vi "RT Main.vi"() -> ()   [LabVIEW 2015]
doc: "The top-level VI for the RIO Eval Kit.\n\nThis VI runs through multiple stages. Each stage demonstrates different features of the RIO Eval Kit. The program uses a \"Queued Message Handler\" architecture. The top loop reads and writes information to and from the FPGA. That information is sent to the bottom through a queue. The information being transfered includes both the data and the type of message being sent. The bottom loop then handles displaying the appropriate information on the LCD."
uses:
  controls/SystemStates.ctl
  <vilib>/EmbeddedDisplay/Hitachi HD44780/Common/Control/screen size.ctl
  <vilib>/EmbeddedDisplay/Hitachi HD44780/Common/Control/font configuration.ctl
  controls/Queue Data.ctl
  controls/SoundOptions.ctl
  <vilib>/FPGAPlugInAG/sbRIO-9637/niLvFpga_Open_sbRIO-9637.vi
  <vilib>/rvi/interface/common/dynamic/niFpgaDynamicAddResources.vi
  <vilib>/Utility/error.llb/Error Cluster From Error Code.vi
  <vilib>/rvi/errors/niLvFpgaAdjustHostInterfaceError.vi
  <vilib>/FPGAPlugInAG/Dynamic/niLvFpga_Close_Dynamic.vi
  <vilib>/rvi/interface/nirviOpenFPGA/nirviOpenFPGA.xnode
  FPGA Bitfiles/LabVIEWRIOEvalua_FPGATarget_FPGA_fRdPegB0rcM.lvbitx
  <vilib>/rvi/interface/nirviMethod/nirviMethod.xnode
  <vilib>/rvi/interface/nirviReadWriteControl/nirviReadWriteControl.xnode
  <vilib>/rvi/interface/nirviCloseFPGA/nirviCloseFPGA.xnode
  <vilib>/EmbeddedDisplay/Hitachi HD44780/Host/HD44780 Host.lvlib
  <vilib>/EmbeddedDisplay/Hitachi HD44780/Common/HD44780 Common.lvlib
  NiFpgaLv.dll
  <vilib>/rvi/interface/Simulation/niFpgaSimulationCallBeginRW.vi
  <vilib>/FPGAPlugInAG/Dynamic/niLvFpga_ReadFifo_Dynamic.vi
  <vilib>/rvi/errors/niLvFpgaMergeErrorWithErrorCode.vi
  usr/local/lib/libamplitude.dll
panel:
  out "Signal":dbl[](graph)
  out "Alarm":bool
  in  "Alarm Threshold":dbl=4.0
  out "Amplitude":dbl format="%#_3g"
  # "Start by turning encoder right to kickoff first stage, and \ncontinue turning right to complete all three stages. Stop \nthe program at any time by pressing the right button (PB2)."
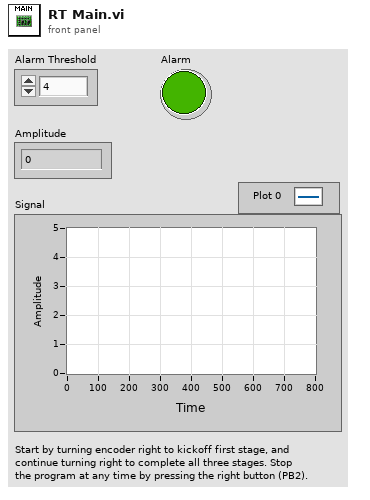
[diagram p1: front panel]
types:
  T1 = typedef "Queue Data.ctl" = cluster{"Current Pos > Threshold?":bool, "Current Pos > Previous?":bool, "Amplitude":dbl, "Stage Number":string}
  T2 = typedef "HD44780 Common.lvlib/font configuration.ctl" = enum8{"5x8 & 2 lines", "5x10 & 1 line", "5x8 & 1 line"}
  T3 = typedef "HD44780 Common.lvlib/screen size.ctl" = enum8{"8x1", "8x2", "12x4", "16x1", "16x2", "16x4", "20x1", "20x2", "20x4", "24x1", "24x2", "40x2", "40x4"}
  T4 = typedef "SystemStates.ctl" = enum16{"Shutdown", "Stage 1", "Stage 2", "Stage 3", "Alarm State"}
  T5 = typedef "SoundOptions.ctl" = enum16{"Ding", "Boing", "Buzzer", "Horn"}
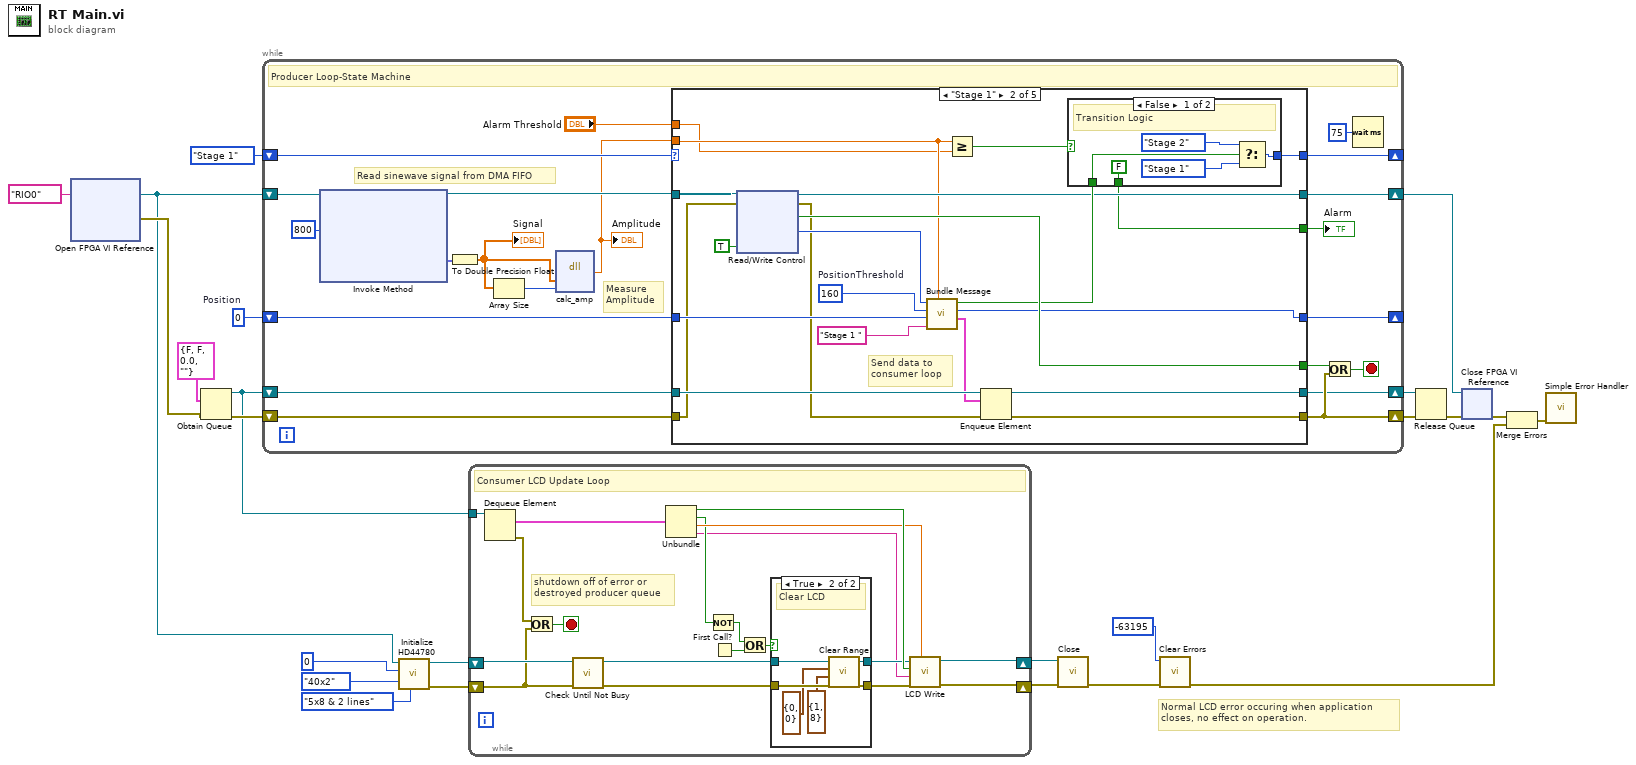
[diagram p0: block diagram]
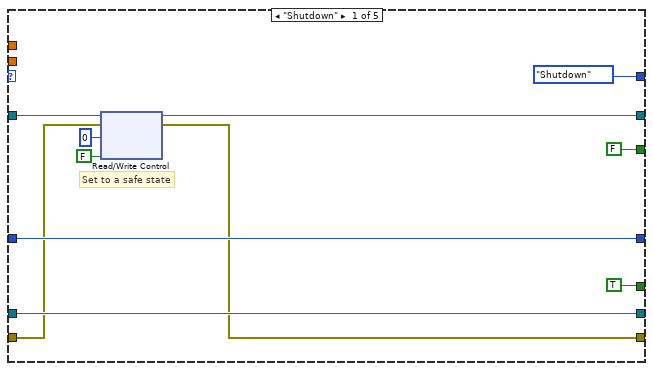
[diagram p3: hidden frame]
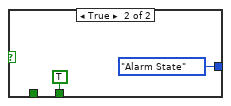
[diagram p4: hidden frame]
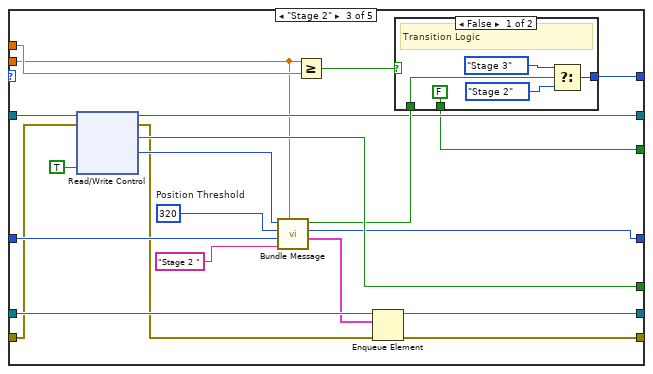
[diagram p5: hidden frame]
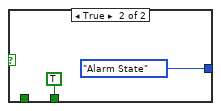
[diagram p6: hidden frame]
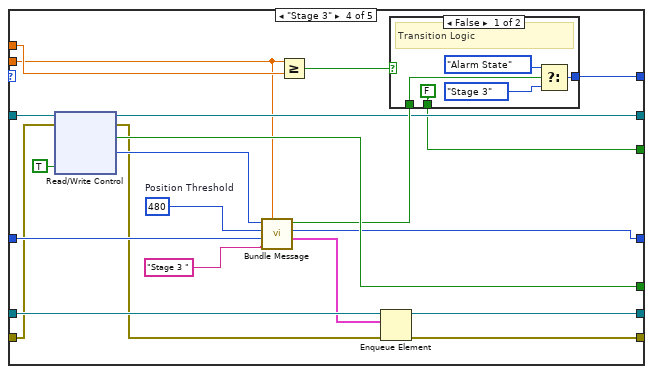
[diagram p7: hidden frame]
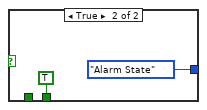
[diagram p8: hidden frame]
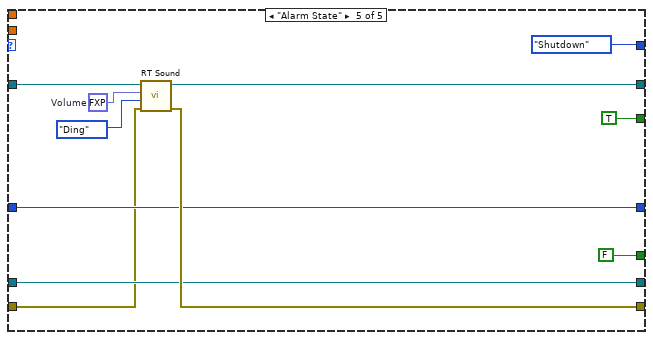
[diagram p9: hidden frame]
diagram:
  w4 = i16 0  # Position
  # "Normal LCD error occuring when application\ncloses, no effect on operation."
  n1 = xnode "Open FPGA VI Reference"("resource name"=tag "RIO0") -> ("FPGA VI Reference Out"=w6:refnum<k20>, "error out"=w10:errorcluster)  [unwired: 1 in]
  n2 = Obtain Queue(element data type=T1 {"Current Pos > Threshold?"=FALSE, "Current Pos > Previous?"=FALSE, "Amplitude"=0.0, "Stage Number"=""} ("output to queue"), error in (no error)=w10) -> (queue out=w7:refnum<queue>, error out=w9:errorcluster)  [unwired: 3 in, 1 out]
  n3 = while {
    shift-right: [w39] -> w23
    shift-left: w9 -> [w28]
    shift-right: [w37] -> w24
    shift-left: w7 -> [w45]
    shift-right: [w41] -> _
    shift-left: SystemStates."Stage 1" ("Enum") -> [w42]
    shift-right: [w29] -> _
    shift-left: w4 -> [w40]
    shift-right: [w36] -> w5
    shift-left: w6 -> [w34]
    stop <- w43 stop-if-true
    # "Measure\nAmplitude"
    # "Read sinewave signal from DMA FIFO"
    # "Producer Loop-State Machine"
    n4 = xnode "Invoke Method"("FPGA VI Reference In"=w34, "Number of Elements"=u32 800) -> ("FPGA VI Reference Out"=w32:refnum<k20>, "Data"=w35:fxp<+/-,24,5>[])  [unwired: 2 in, 2 out]
    n5 = To Double Precision Float(number=w35) -> (double precision float=w26:dbl[])
    "Signal" <- w26
    n6 = Array Size(array=w26) -> (size(s)=w27:i32)
    n7 = dll-call lib="usr/local/lib/libamplitude.*" fn="calc_amp"("waveform"=w26, "length"=w27) -> ("return type"=w25:dbl)  [unwired: 5 in, 2 out]
    "Amplitude" <- w25
    n8 = case shown="\"Stage 1\"" w42 {
      tunnel: w45 -> [w49 w77 w105 w133 w147]
      tunnel: [w48 w76 w104 w132 w151] -> w39
      tunnel: [TRUE w75 w103 w131 FALSE ("E-Stop")] -> w38
      tunnel: [SystemStates."Shutdown" ("Enum") w74 w102 w130 SystemStates."Shutdown" ("Enum")] -> w41
      tunnel: w40 -> [w50 w61 w89 w117 w143]
      tunnel: [w49 w68 w96 w124 w147] -> w37
      tunnel: w32 -> [w53 w67 w95 w123 w142]
      tunnel: [w52 w66 w94 w122 w146] -> w36
      tunnel: w25 -> [_ w63 w92 w120 _]
      tunnel: [FALSE w64 w90 w118 TRUE] -> w31
      tunnel: "Alarm Threshold" -> [_ w62 w93 w121 _]
      tunnel: [w50 w60 w88 w116 w143] -> w29
      tunnel: w28 -> [w47 w57 w85 w113 w141]
      frame "Shutdown" {
        # "Set to a safe state"
        n9 = xnode "Read/Write Control"("FPGA VI Reference In"=w53, "error in"=w47, "Position"=i16 0, "PWM"=FALSE) -> ("FPGA VI Reference Out"=w52:refnum<k20>, "error out"=w48:errorcluster)
      }
      frame "Stage 1" {
        w70 = i16 160  # PositionThreshold
        # "Send data to\nconsumer loop"
        n10 = xnode "Read/Write Control"("FPGA VI Reference In"=w67, "error in"=w57, "PWM"=TRUE) -> ("FPGA VI Reference Out"=w66:refnum<k20>, "error out"=w58:errorcluster, "E-Stop"=w75:bool, "Position"=w69:i16)
        n11 = call "Bundle Message.vi"("Amplitude"=w63, "Stage Number"="Stage 1 " ("text"), "Previous Position"=w61, "Position Threshold"=w70, "Current Position"=w69) -> ("Output to queue"=w59:T1, "Output Position"=w60:i16, "Transition?"=w72:bool)  [unwired: 4 in]
        n12 = Greater Or Equal?(x=w63, y=w62) -> (x >= y?=w65:bool)
        n13 = Enqueue Element(queue=w77, element=w59, error in (no error)=w58) -> (queue out=w68:refnum<queue>, error out=w76:errorcluster)  [unwired: 1 in, 1 out]
        n14 = case shown="False" w65 {
          tunnel: [w80 SystemStates."Alarm State" ("Enum")] -> w74
          tunnel: w72 -> [w79 _]
          tunnel: [FALSE TRUE] -> w64
          frame False {
            # "Transition Logic"
            n15 = Select(t=SystemStates."Stage 2" ("Enum"), s=w79, f=SystemStates."Stage 1" ("Enum")) -> (s? t:f=w80:T4)
          }
          frame True {
          }
        }
      }
      frame "Stage 2" {
        w98 = i16 320  # Position Threshold
        n16 = xnode "Read/Write Control"("FPGA VI Reference In"=w95, "error in"=w85, "PWM"=TRUE) -> ("FPGA VI Reference Out"=w94:refnum<k20>, "error out"=w86:errorcluster, "E-Stop"=w103:bool, "Position"=w97:i16)
        n17 = call "Bundle Message.vi"("Amplitude"=w92, "Stage Number"="Stage 2 " ("text"), "Previous Position"=w89, "Position Threshold"=w98, "Current Position"=w97) -> ("Output to queue"=w87:T1, "Output Position"=w88:i16, "Transition?"=w99:bool)  [unwired: 4 in]
        n18 = Greater Or Equal?(x=w92, y=w93) -> (x >= y?=w91:bool)
        n19 = Enqueue Element(queue=w105, element=w87, error in (no error)=w86) -> (queue out=w96:refnum<queue>, error out=w104:errorcluster)  [unwired: 1 in, 1 out]
        n20 = case shown="False" w91 {
          tunnel: [w108 SystemStates."Alarm State" ("Enum")] -> w102
          tunnel: w99 -> [w107 _]
          tunnel: [FALSE TRUE] -> w90
          frame False {
            # "Transition Logic"
            n21 = Select(t=SystemStates."Stage 3" ("Enum"), s=w107, f=SystemStates."Stage 2" ("Enum")) -> (s? t:f=w108:T4)
          }
          frame True {
          }
        }
      }
      frame "Stage 3" {
        w125 = i16 480  # Position Threshold
        n22 = xnode "Read/Write Control"("FPGA VI Reference In"=w123, "error in"=w113, "PWM"=TRUE) -> ("FPGA VI Reference Out"=w122:refnum<k20>, "error out"=w114:errorcluster, "E-Stop"=w131:bool, "Position"=w126:i16)
        n23 = call "Bundle Message.vi"("Amplitude"=w120, "Stage Number"="Stage 3 " ("text"), "Previous Position"=w117, "Position Threshold"=w125, "Current Position"=w126) -> ("Output to queue"=w115:T1, "Output Position"=w116:i16, "Transition?"=w127:bool)  [unwired: 4 in]
        n24 = Greater Or Equal?(x=w120, y=w121) -> (x >= y?=w119:bool)
        n25 = Enqueue Element(queue=w133, element=w115, error in (no error)=w114) -> (queue out=w124:refnum<queue>, error out=w132:errorcluster)  [unwired: 1 in, 1 out]
        n26 = case shown="False" w119 {
          tunnel: [w136 SystemStates."Alarm State" ("Enum")] -> w130
          tunnel: w127 -> [w135 _]
          tunnel: [FALSE TRUE] -> w118
          frame False {
            # "Transition Logic"
            n27 = Select(t=SystemStates."Alarm State" ("Enum"), s=w135, f=SystemStates."Stage 3" ("Enum")) -> (s? t:f=w136:T4)
          }
          frame True {
          }
        }
      }
      frame "Alarm State" {
        w149 = fxp<+/-,32,16> 5.0  # Volume
        n28 = call "RT Sound.vi"("error in"=w141, "Sound Options"=SoundOptions."Ding" ("Enum"), "Volume"=w149, "FPGA VI Reference In"=w142) -> ("error out"=w151:errorcluster, "FPGA VI Reference Out"=w146:refnum<k20>)  [unwired: 6 in]
      }
    }
    "Alarm" <- w31
    n29 = Or(x=w38, y=w39) -> (x .or. y?=w43:bool)
    n30 = Wait (ms)(milliseconds to wait=u32 75) -> ()  [unwired: 1 out]
  }
  n31 = call <vilib>:"Initialize HD44780.vi"("font configuration (5x8 & 2 lines)"=font_configuration."5x8 & 2 lines", "screen size"=screen_size."40x2", "device index"=i8 0, "FPGA VI Reference in"=w6) -> ("error out"=w16:errorcluster, "LCD out"=w17:refnum<class "Character LCD.lvclass">)  [unwired: 6 in]
  n32 = while {
    shift-right: [w154] -> w15
    shift-left: w17 -> [w170]
    shift-right: [w153] -> w14
    shift-left: w16 -> [w169]
    tunnel: w7 -> [w168]
    stop <- w162 stop-if-true
    # "shutdown off of error or \ndestroyed producer queue"
    # "Consumer LCD Update Loop"
    n33 = Dequeue Element(queue=w168) -> (element=w165:T1, error out=w166:errorcluster)  [unwired: 2 in, 2 out]
    n34 = Or(x=w166, y=w169) -> (x .or. y?=w162:bool)
    n35 = call "Check Until Not Busy.vi"("error in"=w169, "LCD in"=w170) -> ("error out"=w163:errorcluster, "LCD out"=w164:refnum<class "Character LCD.lvclass">)  [unwired: 8 in]
    n36 = Unbundle(w165) -> ("Current Pos > Threshold?"=w167:bool, "Current Pos > Previous?"=w158:bool, "Amplitude"=w161:dbl, "Stage Number"=w152:string)
    n37 = Not(x=w158) -> (.not. x?=w155:bool)
    n38 = First Call?() -> (First Call?: T/F=w156:bool)
    n39 = Or(x=w155, y=w156) -> (x .or. y?=w157:bool)
    n40 = case shown="True" w157 {
      tunnel: w164 -> [w172 w178]
      tunnel: w163 -> [w171 w177]
      tunnel: [w171 w176] -> w159
      tunnel: [w172 w175] -> w160
      frame False {
      }
      frame True {
        # "Clear LCD"
        n41 = call <vilib>:"Clear Range.vi"("error in (no error)"=w177, "end position (end of line)"=cluster{"row":i8, "column":i8} {"row"=1, "column"=8} ("start position"), "start position"=cluster{"row":i8, "column":i8} {"row"=0, "column"=0}, "LCD in"=w178) -> ("error out"=w176:errorcluster, "LCD out"=w175:refnum<class "Character LCD.lvclass">)  [unwired: 6 in]
      }
    }
    n42 = call "LCD Write.vi"("Amplitude"=w161, "error in (no error)"=w159, "Stage Number"=w152, "Current Pos > Threshold?"=w167, "Character LCD in"=w160) -> ("error out"=w153:errorcluster, "LCD out"=w154:refnum<class "Character LCD.lvclass">)  [unwired: 4 in]
  }
  n43 = call <vilib>:"Close.vi"("error in (no error)"=w14, "LCD in"=w15) -> ("error out"=w1:errorcluster)  [unwired: 9 in]
  n44 = call <vilib>:"Clear Errors.vi"("error in (no error)"=w1, "specific error code to clear (0: all)"=-63195) -> ("error out"=w3:errorcluster)  [unwired: 4 in, 1 out]
  n45 = Release Queue(queue=w24, error in (no error)=w23) -> (error out=w22:errorcluster)  [unwired: 1 in, 2 out]
  n46 = xnode "Close FPGA VI Reference"("FPGA VI Reference In"=w5, "error in"=w22) -> ("error out"=w21:errorcluster)
  n47 = Merge Errors(w21, w3) -> (w13:errorcluster)
  n48 = call <vilib>:"Simple Error Handler.vi"("error in (no error)"=w13) -> ()  [unwired: 4 in, 5 out]
